vi "State_Machine.vi"(8 "error in (no error)":errorcluster caption="entrée d'erreur (pas d'erreur)", 11 "Nodon_Get_BP_Status IN":refnum<class "Nodon_Get_BP_Status.lvclass">) -> (0 "error out":errorcluster caption="sortie d'erreur", 2 "Json_String":string, 3 "Nodon_Get_BP_Status OUT":refnum<class "Nodon_Get_BP_Status.lvclass">)   [LabVIEW 2020, in "Library Test.lvlib" / "Nodon_Get_BP_Status.lvclass"]
uses:
  Nodon_Get_BP_Status.lvclass
  C:/Users/ngarcin/OneDrive - Altyor/Standard TB/Class/Test/Nodon_Send_Command_UART/Nodon_Send_Command_UART.lvclass
  Nodon_Send_Command_UART.lvclass
  Nodon_Get_BP_Status.lvclass/Nodon_Get_BP_Status.ctl
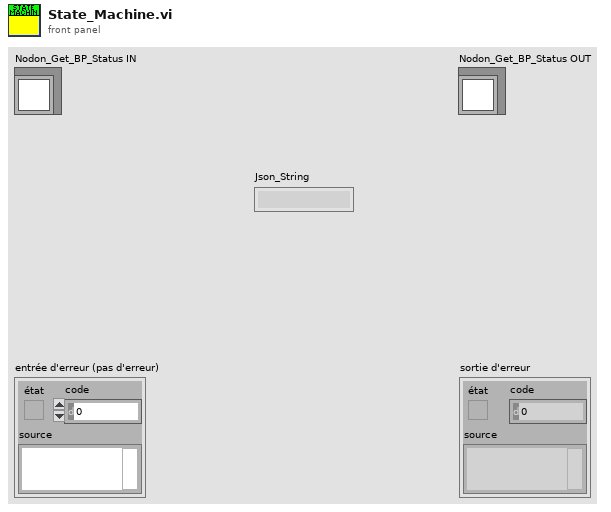
[diagram p1: front panel]
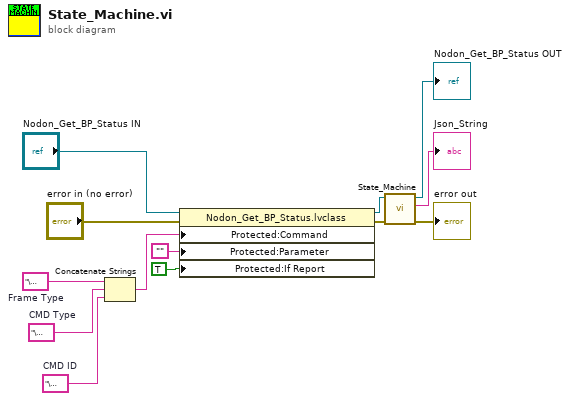
[diagram p0: block diagram]
diagram:
  w5 = "\u0000"  # Frame Type
  w4 = "\u0004"  # CMD ID
  w3 = "\u0001"  # CMD Type
  n1 = Concatenate Strings(w5, w3, w4) -> (w2:string)
  n2 = property class="Nodon_Get_BP_Status.lvclass"(reference="Nodon_Get_BP_Status IN", error in="error in (no error)", "Protected:Command"=w2, "Protected:Parameter"="", "Protected:If Report"=TRUE ("If Report")) -> (reference out=w8:refnum<class "Nodon_Get_BP_Status.lvclass">, error out=w6:errorcluster)
  n3 = call-parent "State_Machine.vi"("error in (no error)"=w6, "Send_Frame en entrée"=w8) -> ("error out"=→"error out":errorcluster, "Json_String"=→"Json_String":string, "Send_Frame en sortie"=→"Nodon_Get_BP_Status OUT":refnum<class "Nodon_Get_BP_Status.lvclass">)  [unwired: 7 in]
